vi "FastArraySumI8.vi"(4 "2-D data array":i8[][](array[numeric]), 6 "sample rate MHz":u16, 7 "Type of Mean":T2=enum."No mean", 8 "Bit Depth":i32=8, 9 "Perform Sum?":bool=TRUE, 10 "Filter Prams":T1, 11 "Data Value Reference in":refnum<data-value>) -> (3 "Data Value Reference out":refnum<data-value>)   [LabVIEW 2022 SP3]
uses:
  ViewData/-ReadEye/TypeDefs/TypeofMean.ctl
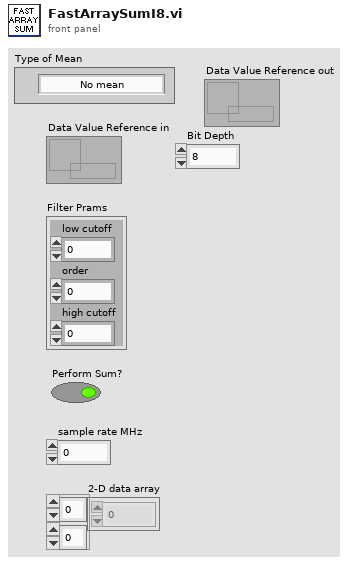
[diagram p1: front panel]
types:
  T1 = cluster{"low cutoff":i32, "order":i32, "high cutoff":i32}
  T2 = typedef "TypeofMean.ctl" = enum16{"Mean from lines", "Mean just lines", "Poly Mean", "No mean", "Filter"}
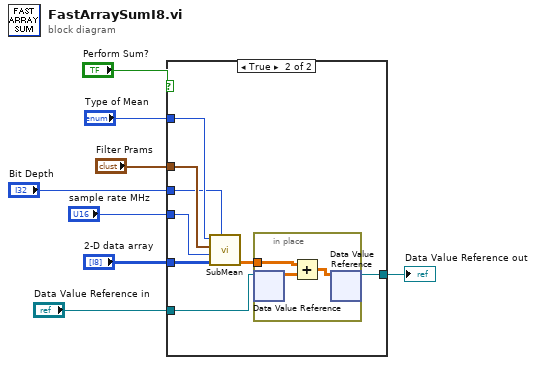
[diagram p0: block diagram]
diagram:
  n1 = case shown="True" "Perform Sum?" {
    tunnel: "Type of Mean" -> [_ w16]
    tunnel: "Filter Prams" -> [_ w15]
    tunnel: "Data Value Reference in" -> [w9 w14]
    tunnel: [w9 w13] -> w4
    tunnel: "2-D data array" -> [_ w12]
    tunnel: "sample rate MHz" -> [_ w11]
    tunnel: "Bit Depth" -> [_ w10]
    frame False {
    }
    frame True {
      n2 = call "SubMean.vi"("Bit Depth"=w10, "Scan Data In"=w12, "Samp Rate (MHz)"=w11, "Filter Prams"=w15, "Type of Mean"=w16) -> ("Array"=w17:dbl[][])  [unwired: 1 in, 2 out]
      n3 = in-place {
        in-place-border: w17 -> [w18]
        n4 = in-place-dvr #1(w14) -> (w20:dbl[][])  [unwired: 1 out]
        n5 = Add(x=w18, y=w20) -> (x+y=w19:dbl[][])
        n6 = in-place-dvr #1(w19) -> (w13:refnum<data-value>)  [unwired: 1 out]
      }
    }
  }
  "Data Value Reference out" <- w4
